vi "Build Tree Struct wProperties.vi"(8 "error in":errorcluster, 10 "VIs (including clones)":string[](array[string]), 11 "ConfigInfo in":T1={"Data Tree Ref"=refnum, "FP Ref"=refnum, "Column Data Type"=[], "Search Clones Up To"=100, "SortOptions"={"Col.pri"=0, "RevDir.pri"=FALSE, "Col.sec"=0, "RevDir.sec"=FALSE}, "Group/Flat (0:group)"=FALSE, "CollapsedNodes"=[], "Show/Hide Cols"=[], "Filtered Paths"=[], "View"=enum."Group By Library", "File Extension Filters"=[], "Filter Global VIs"=FALSE, "Shared"=refnum}) -> (0 "error out":errorcluster, 1 "Canceled":bool)   [LabVIEW 2013, in "LVTM.lvlib"]
uses:
  LVTM.lvlib
  Controls_LVTM/LVTM_Config_Info.ctl
  Controls_LVTM/View.ctl
  Controls_LVTM/SharedDataDVR.ctl
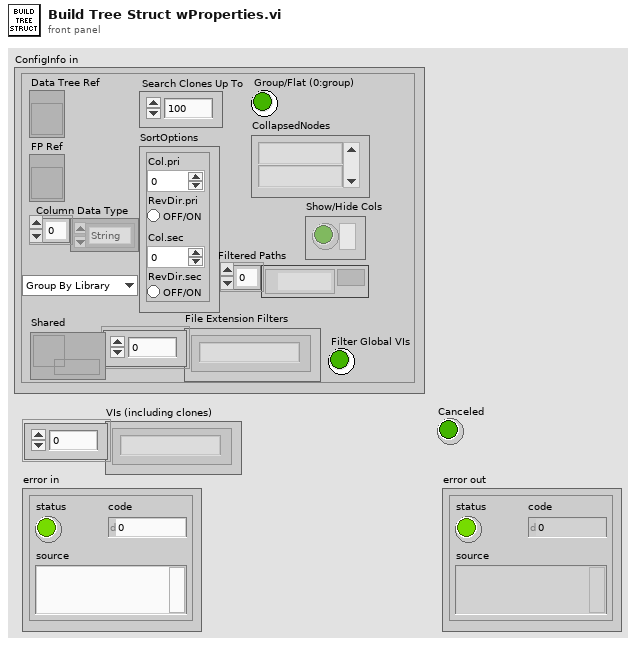
[diagram p1: front panel]
types:
  T1 = typedef "LVTM.lvlib/LVTM_Config_Info.ctl" = cluster{"Data Tree Ref":refnum<vi>, "FP Ref":refnum<vi>, "Column Data Type":enum16{"String", "Numeric"}[], "Search Clones Up To":i32, "SortOptions":cluster{"Col.pri":i32, "RevDir.pri":bool, "Col.sec":i32, "RevDir.sec":bool}, "Group/Flat (0:group)":bool, "CollapsedNodes":string[], "Show/Hide Cols":bool[], "Filtered Paths":path[], "View":T2, "File Extension Filters":string[], "Filter Global VIs":bool, "Shared":refnum<data-value>}
  T2 = typedef "LVTM.lvlib/View.ctl" = enum16{"Group By Library", "Group By Folder", "Flat List"}
  T3 = typedef "LVTM.lvlib/SharedDataDVR.ctl" = cluster{"App":refnum<vi>, "VIs":string[]}
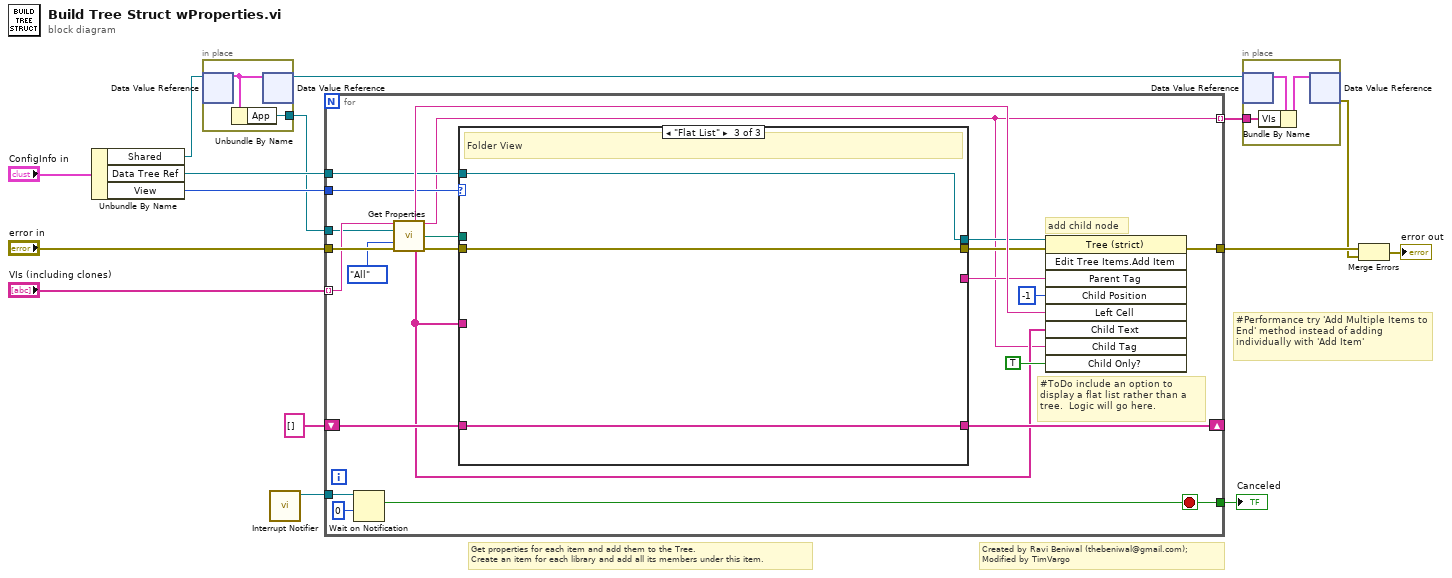
[diagram p0: block diagram]
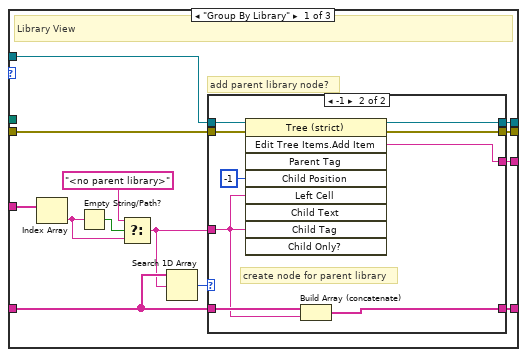
[diagram p2: hidden frame]
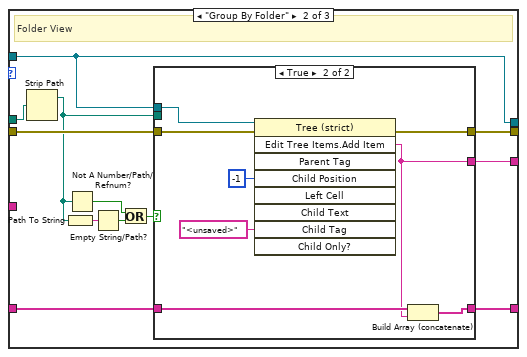
[diagram p4: hidden frame]
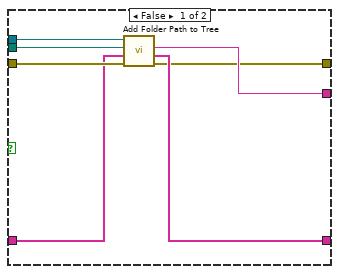
[diagram p5: hidden frame]
diagram:
  # "Created by Ravi Beniwal (thebeniwal@gmail.com);\nModified by TimVargo"
  # "#Performance try 'Add Multiple Items to End' method instead of adding individually with 'Add Item'"
  # "Get properties for each item and add them to the Tree.\nCreate an item for each library and add all its members under this item."
  n1 = Unbundle By Name("ConfigInfo in") -> ("Shared"=w8:refnum<data-value>, "Data Tree Ref"=w15:refnum<vi>, "View"=w10:T2)
  n2 = in-place {
    in-place-border: [w16] -> w7
    n3 = in-place-dvr #1(w8) -> (w17:T3)  [unwired: 1 out]
    n4 = Unbundle By Name(w17) -> ("App"=w16:refnum<vi>)
    n5 = in-place-dvr #1(w17) -> (w6:refnum<data-value>)  [unwired: 1 out]
  }
  n6 = call "Interrupt Notifier.vi"() -> ("Notifier out"=w2:refnum<notifier>)  [unwired: 10 in, 1 out]
  n7 = for {
    tunnel: "VIs (including clones)" -> [w36] mode=indexing
    tunnel: "error in" -> [w38]
    tunnel: [w37] -> w14
    tunnel: w7 -> [w34]
    shift-right: [w30] -> _
    shift-left: string[] [] -> [w31]
    tunnel: w15 -> [w29]
    tunnel: w10 -> [w23]
    tunnel: [w21] -> w5 mode=indexing
    tunnel: w2 -> [w19]
    tunnel: [w18] -> w1
    stop <- w18 stop-if-true
    # "#ToDo include an option to display a flat list rather than a tree.  Logic will go here."
    # "add child node"
    n8 = Wait on Notification(notifier=w19, timeout in ms (-1)=0) -> (notification=w18:bool)  [unwired: 2 in, 3 out]
    n9 = call "Get Properties.vi"("VI Name"=w36, "AppInst"=w34, "Scope (0:All)"=enum16{"All", "Dynamic"}."All", "error in"=w38) -> ("File Name Out"=w35:string, "Full Name Out"=w21:string, "Path"=w22:path, "VI Properties (All)"=w25:string[], "error out"=w32:errorcluster)  [unwired: 3 in, 4 out]
    n10 = case shown="\"Flat List\"" w23 {
      tunnel: [w52 w72 w94] -> w33
      tunnel: w32 -> [w51 w76 w94]
      tunnel: w31 -> [w50 w74 w93]
      tunnel: [w49 w73 w93] -> w30
      tunnel: w29 -> [w48 w71 w95]
      tunnel: [w47 w71 w95] -> w28
      tunnel: [w46 w75 _] -> w26
      tunnel: w25 -> [w44 _ _]
      tunnel: w22 -> [_ w77 _]
      frame "Group By Library" {
        # "add parent library node?"
        # "Library View"
        n11 = Index Array(array=w44) -> (element=w41:string)  [unwired: 1 in]
        n12 = Empty String/Path?(string/path=w41) -> (empty?=w42:bool)
        n13 = Select(t="<no parent library>", s=w42, f=w41) -> (s? t:f=w43:string)
        n14 = Search 1D Array(1D array=w50, element=w43) -> (index of element=w45:i32)  [unwired: 1 in]
        n15 = case shown="-1" w45 {
          tunnel: [w55 w64] -> w52
          tunnel: w51 -> [w55 w63]
          tunnel: [w54 w62] -> w49
          tunnel: w50 -> [w54 w61]
          tunnel: w43 -> [w53 w57]
          tunnel: w48 -> [w56 w60]
          tunnel: [w56 w59] -> w47
          tunnel: [w53 w58] -> w46
          frame 0, Default {
            # "parent library already exists"
          }
          frame -1 {
            # "create node for parent library"
            n16 = invoke on="Invoke Node" class="Tree (strict)" method="Edit Tree Items.Add Item"(reference=w60, error in=w63, "Child Position"=-1, "Left Cell"=w57, "Child Tag"=w57) -> (reference out=w59:refnum<vi>, error out=w64:errorcluster, "Edit Tree Items:Add Item"=w58:string)  [unwired: 4 in, 6 out]
            n17 = Build Array (concatenate)(w61, w57) -> (w62:string[])
          }
        }
      }
      frame "Group By Folder" {
        # "Folder View"
        n18 = Strip Path(path=w77) -> (stripped path=w67:path)  [unwired: 1 out]
        n19 = Path To String(path=w67) -> (string=w68:string)
        n20 = Not A Number/Path/Refnum?(number/path/refnum=w67) -> (NaN/Path/Refnum?=w70:bool)
        n21 = Empty String/Path?(string/path=w68) -> (empty?=w69:bool)
        n22 = Or(x=w70, y=w69) -> (x .or. y?=w66:bool)
        n23 = case shown="True" w66 {
          tunnel: w76 -> [w84 w90]
          tunnel: [w83 w85] -> w75
          tunnel: w74 -> [w82 w88]
          tunnel: [w81 w87] -> w73
          tunnel: [w80 w86] -> w72
          tunnel: w71 -> [w79 w89]
          tunnel: w67 -> [w78 _]
          frame False {
            n24 = call "Add Folder Path to Tree.vi"("error in (no error)"=w84, "All Folder Tags"=w82, "Folder Path"=w78, "TreeControl in"=w79) -> ("error out"=w80:errorcluster, "All Folder Tags Out"=w81:string[], "Folder Item Tag"=w83:string)  [unwired: 5 in]
          }
          frame True {
            n25 = invoke on="Invoke Node" class="Tree (strict)" method="Edit Tree Items.Add Item"(reference=w89, error in=w90, "Child Position"=-1, "Child Tag"="<unsaved>") -> (error out=w86:errorcluster, "Edit Tree Items:Add Item"=w85:string)  [unwired: 5 in, 7 out]
            n26 = Build Array (concatenate)(w88, w85) -> (w87:string[])
          }
        }
      }
      frame "Flat List" {
        # "Folder View"
      }
    }
    n27 = invoke on="Invoke Node" class="Tree (strict)" method="Edit Tree Items.Add Item"(reference=w28, error in=w33, "Parent Tag"=w26, "Child Position"=-1, "Left Cell"=w35, "Child Text"=w25, "Child Tag"=w21, "Child Only?"=TRUE) -> (error out=w37:errorcluster)  [unwired: 1 in, 8 out]
  }
  "Canceled" <- w1
  n28 = in-place {
    in-place-border: w5 -> [w96]
    n29 = in-place-dvr #2(w6) -> (w98:T3)  [unwired: 1 out]
    n30 = Bundle By Name(cluster=w98, "VIs"=w96) -> (w97:T3)
    n31 = in-place-dvr #2(w97) -> (w3:errorcluster)  [unwired: 1 out]
  }
  n32 = Merge Errors(w14, w3) -> (→"error out":errorcluster)
